vi "Init Base Graph.vi"(6 "Z Scale.Marker Values[]":cluster{"Numeric":dbl, "Numeric":u32}[](array[cluster]), 8 "error in (no error)":errorcluster, 9 "Sizes":cluster{"Height":u32, "Width":u32}, 10 "IntGraph Ref":refnum<vi>, 11 "TG Base Graph in":refnum<class "Base Graph.lvclass">) -> (0 "error out":errorcluster, 3 "TG Base Graph out":refnum<class "Base Graph.lvclass">)   [LabVIEW 2023, in "Base Graph.lvclass"]
uses:
  Base Graph.lvclass
  Base Graph.lvclass/Base Graph.ctl
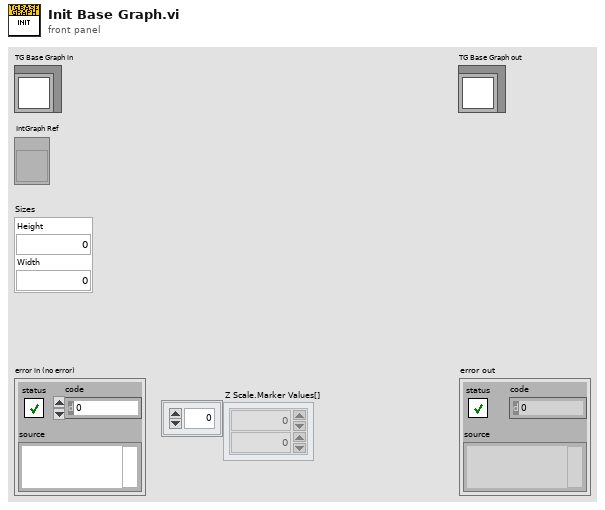
[diagram p1: front panel]
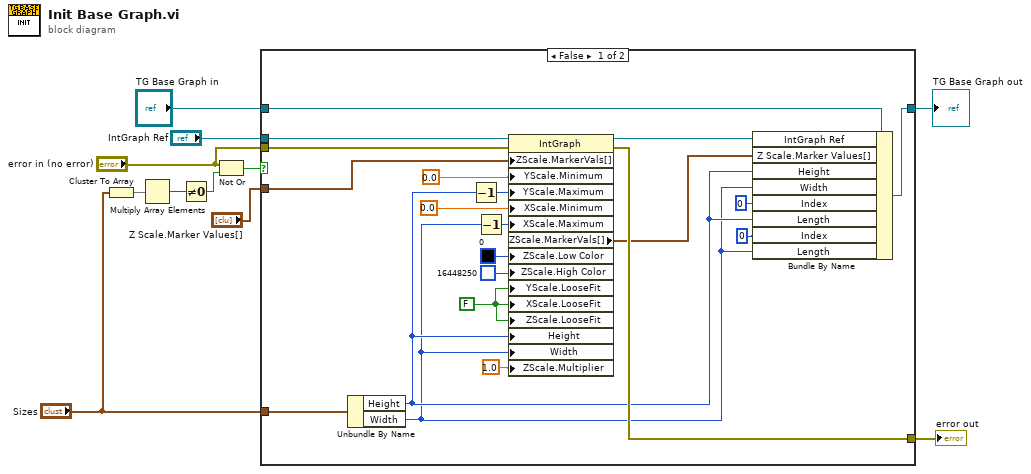
[diagram p0: block diagram]
diagram:
  n1 = Cluster To Array(cluster="Sizes") -> (array=w4:u32[])
  n2 = Multiply Array Elements(1:w4) -> (0:w3:u32)
  n3 = Not Equal To 0?(x=w3) -> (x != 0?=w2:bool)
  n4 = Not Or(1:w2, 2:"error in (no error)") -> (0:w5:bool)
  n5 = case shown="False" w5 {
    tunnel: [w26 w33] -> w11
    tunnel: [w31 w34] -> w9
    tunnel: "TG Base Graph in" -> [w32 w34]
    tunnel: "IntGraph Ref" -> [w30 _]
    tunnel: "Z Scale.Marker Values[]" -> [w28 _]
    tunnel: "Sizes" -> [w27 _]
    tunnel: "error in (no error)" -> [w15 w33]
    frame False {
      w18 = FALSE ("X Scale.Loose Fit")
      n6 = Unbundle By Name(w27) -> ("Height"=w17:u32, "Width"=w16:u32)
      n7 = Decrement(x=w17) -> (x-1=w14:u32)
      n8 = Decrement(x=w16) -> (x-1=w13:u32)
      n9 = property class="IntGraph"(reference=w30, error in=w15, "ZScale.MarkerVals[]"=w28, "YScale.Minimum"=0.0 ("Y Scale.Range:Minimum"), "YScale.Maximum"=w14, "XScale.Minimum"=0.0 ("X Scale.Range:Minimum"), "XScale.Maximum"=w13, "ZScale.Low Color"=u32 0 ("Z Scale.Low Color"), "ZScale.High Color"=u32 16448250 ("Z Scale.High Color"), "YScale.LooseFit"=w18, "XScale.LooseFit"=w18, "ZScale.LooseFit"=w18, "Height"=w17, "Width"=w16, "ZScale.Multiplier"=1.0 ("Z Scale.Offset and Multiplier:Multiplier")) -> (reference out=w29:refnum<vi>, error out=w26:errorcluster, "ZScale.MarkerVals[]"=w23:cluster{dbl, u32}[])
      n10 = Bundle By Name(cluster=w32, "IntGraph Ref"=w29, "Z Scale.Marker Values[]"=w23, "Height"=w17, "Width"=w16, "Index"=u32 0 ("ROI XY.ROI Y.Index"), "Length"=w17, "Index"=u32 0 ("ROI XY.ROI X.Index"), "Length"=w16) -> (w31:refnum<class "Base Graph.lvclass">)
    }
    frame True {
    }
  }
  "error out" <- w11
  "TG Base Graph out" <- w9
